vi "DS18b20 Read.vi"(8 "error in (no error)":errorcluster, 11 "id":string="28-000006ca18d4") -> (0 "error out":errorcluster, 3 "Temp":dbl)   [LabVIEW 2014, in "QwaveSys Raspberry Pi Library.lvlib"]
uses:
  QwaveSys Raspberry Pi Library.lvlib
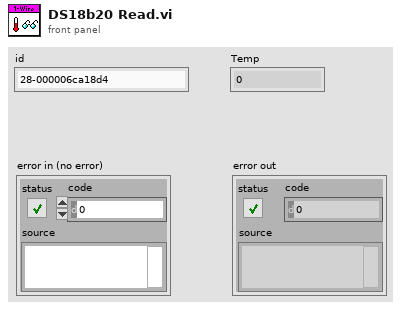
[diagram p1: front panel]
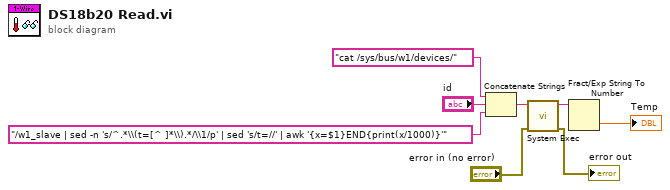
[diagram p0: block diagram]
diagram:
  n1 = Concatenate Strings("cat /sys/bus/w1/devices/" ("command line"), "id", "/w1_slave | sed -n 's/^.*\\(t=[^ ]*\\).*/\\1/p' | sed 's/t=//' | awk '{x=$1}END{print(x/1000)}'" ("command line")) -> (w8:string)
  n2 = call <vilib>:"System Exec.vi"("error in (no error)"="error in (no error)", "command line"=w8) -> ("error out"=→"error out":errorcluster, "standard output"=w4:string)  [unwired: 6 in, 2 out]
  n3 = Fract/Exp String To Number(string=w4) -> (number=→"Temp":dbl)  [unwired: 3 in, 1 out]
